vi "tearDown.vi"(8 "error in (no error)":errorcluster, 11 "reference in":refnum<class "Instrument Addon Common System Tests.lvclass">) -> (0 "error out":errorcluster, 3 "reference out":refnum<class "Instrument Addon Common System Tests.lvclass">)   [LabVIEW 2020, in "Instrument Addon Common System Tests.lvclass"]
doc: "tearDown runs after the test method has completed. Use this method to clean up any operations or references that were opened by setUp or the test method. Unit tests should be independent of other unit tests so this VI should ensure that the next test can run in a 'clean' test environment."
uses:
  Instrument Addon Common System Tests.lvclass
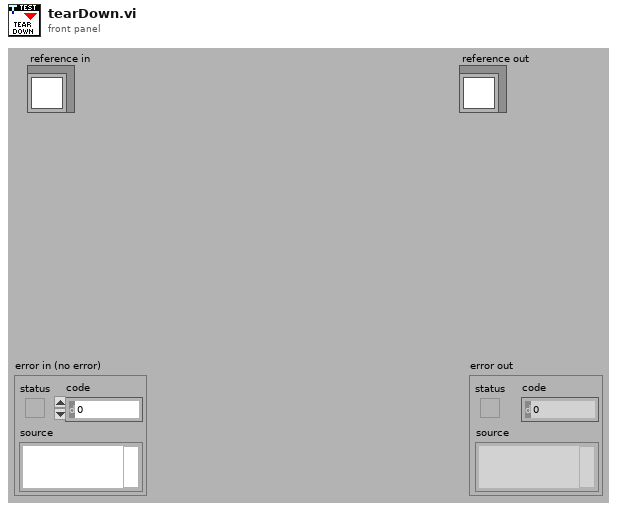
[diagram p1: front panel]
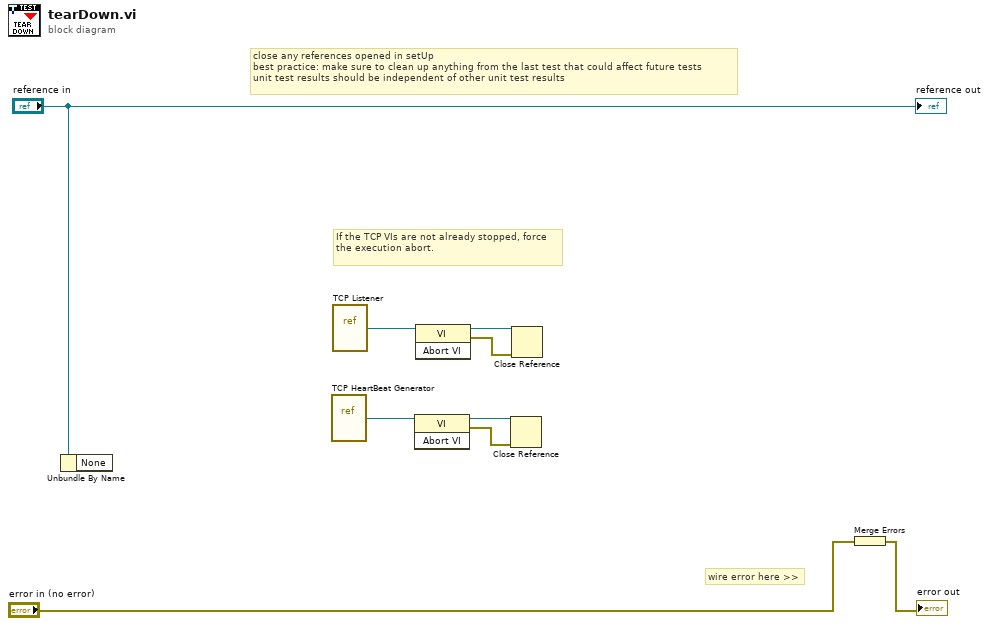
[diagram p0: block diagram]
diagram:
  # "If the TCP VIs are not already stopped, force the execution abort."
  # "wire error here >>"
  # "close any references opened in setUp\nbest practice: make sure to clean up anything from the last test that could affect future tests\nunit test results should be independent of other unit test results"
  n1 = Unbundle By Name("reference in") -> ()  [unwired: 1 out]
  n2 = vi-ref "TCP HeartBeat Generator.vi"() -> (w1:refnum<vi>)
  n3 = vi-ref "TCP Listener.vi"() -> (w7:refnum<vi>)
  n4 = invoke class="VI" method="Abort VI"(reference=w1) -> (reference out=w2:refnum<vi>, error out=w3:errorcluster)  [unwired: 2 in, 1 out]
  n5 = invoke class="VI" method="Abort VI"(reference=w7) -> (reference out=w5:refnum<vi>, error out=w4:errorcluster)  [unwired: 2 in, 1 out]
  n6 = Close Reference(reference=w2, error in (no error)=w3) -> ()  [unwired: 1 out]
  n7 = Close Reference(reference=w5, error in (no error)=w4) -> ()  [unwired: 1 out]
  n8 = Merge Errors("error in (no error)") -> (→"error out":errorcluster)
  "reference out" <- "reference in"
